vi "GE TRIALNEW 25.vi"() -> ()   [LabVIEW 2014]
uses:
  <vilib>/LabVIEW Targets/FPGA/cRIO/shared/nicrio_ModuleControls/nicrio_cRIO-9225_DataRatesRing.ctl
  <vilib>/LabVIEW Targets/FPGA/cRIO/shared/nicrio_ModuleControls/nicrio_cRIO-9227_DataRatesRing.ctl
  <vilib>/rvi/FXPMathLib/FxpSinAndCos/subVIs/nifxpmath_SinAndCos_SimConfig.ctl
  <vilib>/rvi/FXPMathLib/FxpRectToPolar/subVIs/nifxpmath_RectToPolar_SimConfig.ctl
  <vilib>/rvi/FXPMathLib/FxpDiv/subVIs/nifxpmath_Div_SimConfig.ctl
  <vilib>/rvi/Emulation/niFpgaGetClockAttributes.vi
  <vilib>/rvi/Emulation/niFpgaSctlEmulationGetInTimedLoop.vi
  <vilib>/rvi/Emulation/niFpgaEmulationReportErrorSimple.vi
  <vilib>/rvi/eio/common/nirviEmuTemplateMethod_errors.vi
  <vilib>/rvi/Memory/Memory_Emulation/nirvimemoryFastEmulation.vi
  <vilib>/rvi/Memory/Memory_Emulation/nirvimemoryEmulation.vi
  <vilib>/rvi/Emulation/niFpgaEmulationIsFPGAContextNoSignature.vi
  <vilib>/rvi/DataTransferAndStorage/Container/Common/niFpgaContainerGetUniqueNameForEmu.vi
  <vilib>/rvi/Emulation/niFpgaProcessEmulError.vi
  <vilib>/rvi/errors/nirviReportUnexpectedCaseInternalError (U32).vi
  <vilib>/rvi/FXPMathLib/FxpSinAndCos/simVIs/DllFxpSinAndCosTemp_sub.vi
  <vilib>/rvi/FXPMathLib/FxpRectToPolar/simVIs/DllFxpRectToPolarTemp_sub.vi
  <vilib>/rvi/FXPMathLib/FxpDiv/simVIs/DllFxpDivTemp_sub.vi
  <vilib>/rvi/Emulation/niFpgaCriticalErrorInLSC.vi
  <vilib>/rvi/DataTransferAndStorage/Container/Common/niFpgaContainerSetEmuInfo.vi
  <vilib>/rvi/eio/common/nirviEmuReportErrorAndStop.vi
  <vilib>/rvi/eio/common/nirviEmuTemplatePropertySet_noerrors.vi
  <vilib>/eio/EIONode/EIONode.xnode
  <vilib>/rvi/DataTransferAndStorage/Container/XNode/niFpgaContainer.xnode
  <vilib>/rvi/FXPMathLib/FxpSub/XNode/nifxpmath_Sub.xnode
  <vilib>/rvi/FXPMathLib/FxpMul/XNode/nifxpmath_Multiplier.xnode
  <vilib>/rvi/FXPMathLib/FxpSinAndCos/XNode/nifxpmath_SinAndCos.xnode
  <vilib>/rvi/FXPMathLib/FxpAdd/XNode/nifxpmath_Add.xnode
  <vilib>/rvi/FXPMathLib/FxpRectToPolar/XNode/nifxpmath_RectToPolar.xnode
  <vilib>/rvi/FXPMathLib/FxpDiv/XNode/nifxpmath_Div.xnode
  <vilib>/rvi/LocalResourceManager/LocalResourceManager.xnode
  <vilib>/eio/EIOPropertyNode/EIOPropertyNode.xnode
  <vilib>/rvi/FXPMathLib/sim/FxpSim.dll
  <vilib>/rvi/eio/common/nirviEmuTemplatePropertyGet_errors.vi
  <vilib>/rvi/eio/common/nirviEmuTemplatePropertyGet_noerrors.vi
  <vilib>/rvi/eio/common/nirviEmuTemplatePropertySet_errors.vi
panel:
  in  "stop":bool
  out "Angle Actual":fxp<+/-,22,10>[](array[numeric])
  out "Magnitude Actual":fxp<+,52,38>[](array[numeric])
  out "Ym Magnitude":fxp<+/-,64,39>[](array[numeric])
  out "Ym Angle":fxp<+/-,22,10>[](array[numeric])
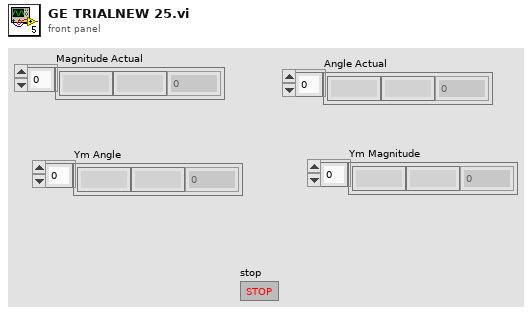
[diagram p1: front panel]
types:
  T1 = typedef "nicrio_cRIO-9227_DataRatesRing.ctl" = u8
  T2 = typedef "nicrio_cRIO-9225_DataRatesRing.ctl" = u8
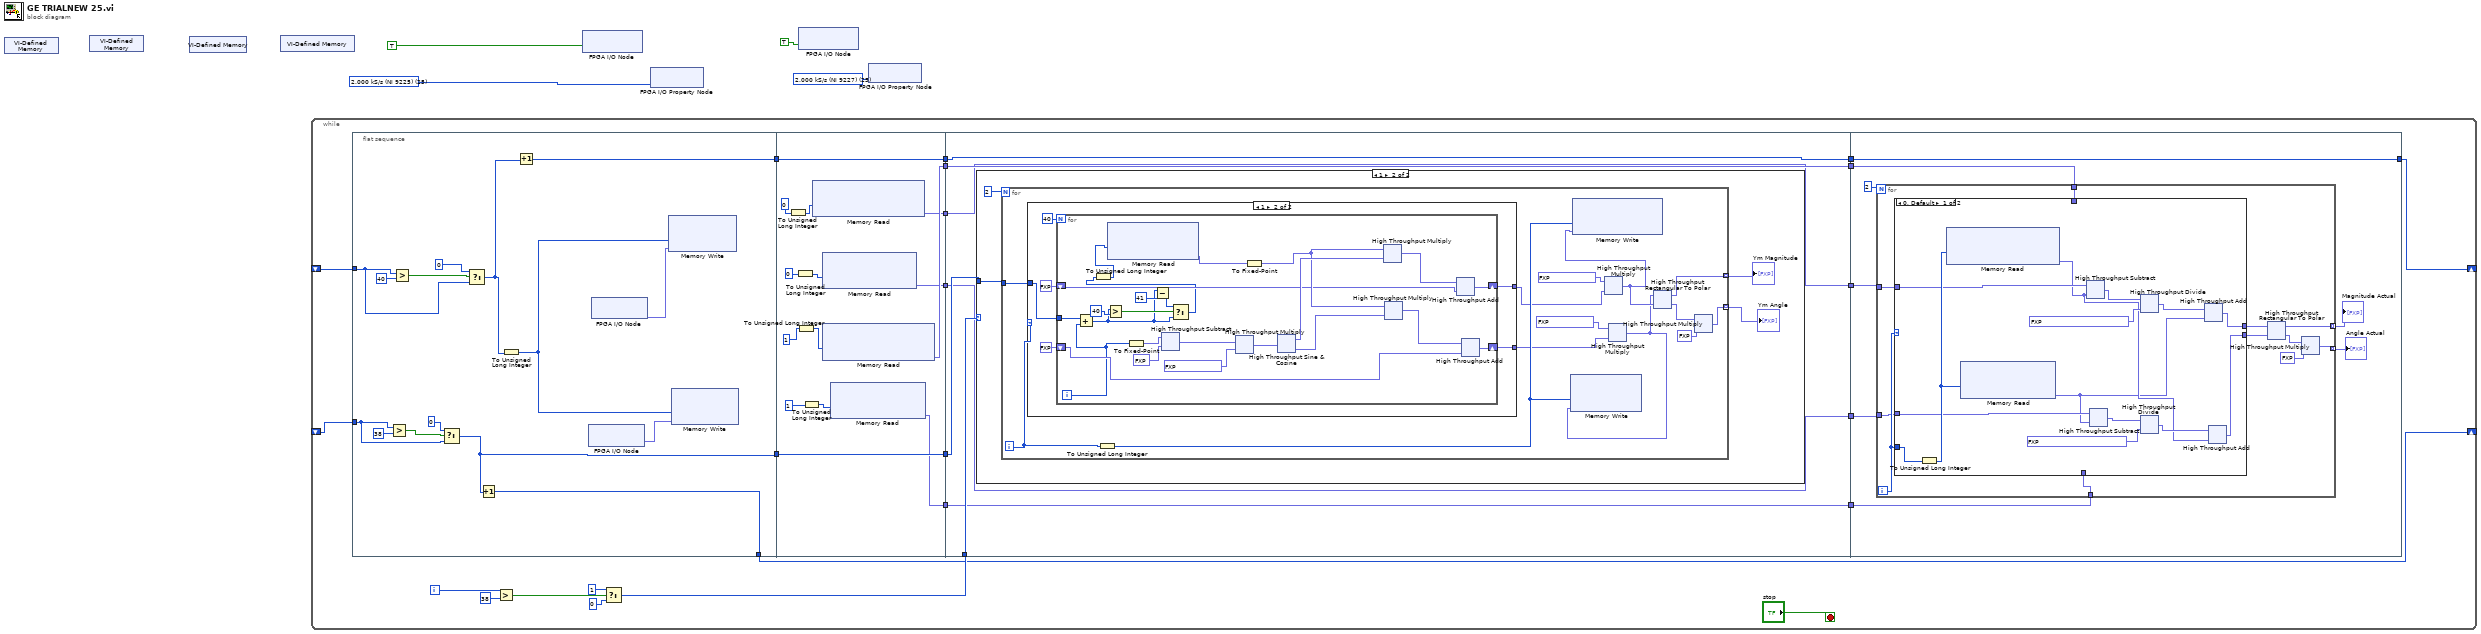
[diagram p0: block diagram]
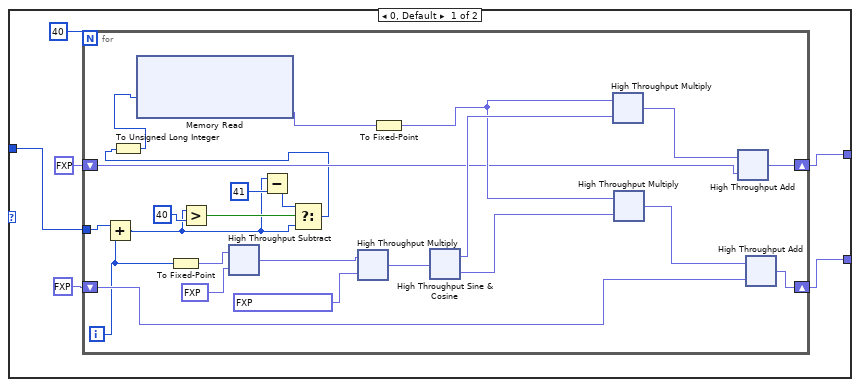
[diagram p3: hidden frame]
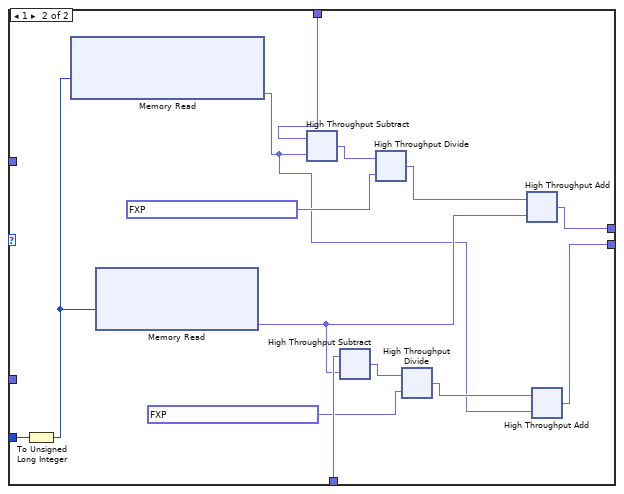
[diagram p4: hidden frame]
diagram:
  w1 = T1 25 items=["50.000 kS/s (NI 9227)"=1, "25.000 kS/s (NI 9227)"=2, "16.667 kS/s (NI 9227)"=3, "12.500 kS/s (NI 9227)"=4, "10.000 kS/s (NI 9227)"=5, "8.333 kS/s (NI 9227)"=6, "7.143 kS/s (NI 9227)"=7, "6.250 kS/s (NI 9227)"=8, "5.556 kS/s (NI 9227)"=9, "5.000 kS/s (NI 9227)"=10, "4.545 kS/s (NI 9227)"=11, "4.167 kS/s (NI 9227)"=12, "3.846 kS/s (NI 9227)"=13, "3.571 kS/s (NI 9227)"=14, "3.333 kS/s (NI 9227)"=15, "3.125 kS/s (NI 9227)"=16, "2.941 kS/s (NI 9227)"=17, "2.778 kS/s (NI 9227)"=18, "2.632 kS/s (NI 9227)"=19, "2.500 kS/s (NI 9227)"=20, "2.381 kS/s (NI 9227)"=21, "2.273 kS/s (NI 9227)"=22, "2.174 kS/s (NI 9227)"=23, "2.083 kS/s (NI 9227)"=24, "2.000 kS/s (NI 9227)"=25, "1.923 kS/s (NI 9227)"=26, "1.852 kS/s (NI 9227)"=27, "1.786 kS/s (NI 9227)"=28, "1.724 kS/s (NI 9227)"=29, "1.667 kS/s (NI 9227)"=30, "1.613 kS/s (NI 9227)"=31] ("Data Rate")
  w2 = T2 25 items=["50.000 kS/s (NI 9225)"=1, "25.000 kS/s (NI 9225)"=2, "16.667 kS/s (NI 9225)"=3, "12.500 kS/s (NI 9225)"=4, "10.000 kS/s (NI 9225)"=5, "8.333 kS/s (NI 9225)"=6, "7.143 kS/s (NI 9225)"=7, "6.250 kS/s (NI 9225)"=8, "5.556 kS/s (NI 9225)"=9, "5.000 kS/s (NI 9225)"=10, "4.545 kS/s (NI 9225)"=11, "4.167 kS/s (NI 9225)"=12, "3.846 kS/s (NI 9225)"=13, "3.571 kS/s (NI 9225)"=14, "3.333 kS/s (NI 9225)"=15, "3.125 kS/s (NI 9225)"=16, "2.941 kS/s (NI 9225)"=17, "2.778 kS/s (NI 9225)"=18, "2.632 kS/s (NI 9225)"=19, "2.500 kS/s (NI 9225)"=20, "2.381 kS/s (NI 9225)"=21, "2.273 kS/s (NI 9225)"=22, "2.174 kS/s (NI 9225)"=23, "2.083 kS/s (NI 9225)"=24, "2.000 kS/s (NI 9225)"=25, "1.923 kS/s (NI 9225)"=26, "1.852 kS/s (NI 9225)"=27, "1.786 kS/s (NI 9225)"=28, "1.724 kS/s (NI 9225)"=29, "1.667 kS/s (NI 9225)"=30, "1.613 kS/s (NI 9225)"=31] ("Data Rate")
  n1 = xnode "VI-Defined Memory"() -> ()  [unwired: 1 out]
  n2 = xnode "VI-Defined Memory"() -> ()  [unwired: 1 out]
  n3 = xnode "VI-Defined Memory"() -> ()  [unwired: 1 out]
  n4 = xnode "VI-Defined Memory"() -> ()  [unwired: 1 out]
  n5 = while {
    shift-right: [w21] -> _
    shift-left: _ -> [w22]
    shift-right: [w18] -> _
    shift-left: _ -> [w19]
    i -> [w25]
    stop <- "stop" stop-if-true
    n6 = flat-sequence {
      tunnel: w22 -> [w35]
      tunnel: [w37] -> w16
      tunnel: w19 -> [w31]
      tunnel: [w30] -> w18
      tunnel: [w29] -> w14
      tunnel: w16 -> [w57]
      tunnel: [w57] -> w15
      tunnel: w14 -> [w56]
      tunnel: [w56] -> w13
      tunnel: [w55] -> w11
      tunnel: [w54] -> w9
      tunnel: [w53] -> w7
      tunnel: [w52] -> w5
      tunnel: w23 -> [w64]
      tunnel: w15 -> [w63]
      tunnel: w13 -> [w62]
      tunnel: [w63] -> w17
      tunnel: [w61] -> w12
      tunnel: w11 -> [w61]
      tunnel: [w60] -> w10
      tunnel: w9 -> [w60]
      tunnel: [w59] -> w8
      tunnel: w7 -> [w59]
      tunnel: [w58] -> w6
      tunnel: w5 -> [w58]
      tunnel: [w246] -> w21
      tunnel: w17 -> [w246]
      tunnel: w12 -> [w244]
      tunnel: w10 -> [w243]
      tunnel: w8 -> [w242]
      tunnel: w6 -> [w241]
      frame #0 {
        n7 = Greater?(x=w31, y=38) -> (0:w32:bool)
        n8 = Greater?(x=w35, y=40) -> (0:w42:bool)
        n9 = Select(t=0, s=w32, f=w31) -> (s? t:f=w29:i32)
        n10 = Select(t=0, s=w42, f=w35) -> (s? t:f=w38:i32)
        n11 = Increment(x=w29) -> (x+1=w30:i32)
        n12 = To Unsigned Long Integer(number=w38) -> (unsigned 32bit integer=w41:u32)
        n13 = Increment(x=w38) -> (x+1=w37:i32)
        n14 = xnode "FPGA I/O Node"() -> ("Mod1/AI0"=w40:fxp<+/-,24,10>)  [unwired: 1 in, 1 out]
        n15 = xnode "FPGA I/O Node"() -> ("Mod2/AI0"=w39:fxp<+/-,24,5>)  [unwired: 1 in, 1 out]
        n16 = xnode ("Memory Write")("Address"=w41, "Data"=w39) -> ()  [unwired: 1 in, 1 out]
        n17 = xnode ("Memory Write")("Address"=w41, "Data"=w40) -> ()  [unwired: 1 in, 1 out]
      }
      frame #1 {
        n18 = To Unsigned Long Integer(number=u32 0 ("Address")) -> (unsigned 32bit integer=w50:u32)
        n19 = To Unsigned Long Integer(number=u32 0 ("Address")) -> (unsigned 32bit integer=w48:u32)
        n20 = To Unsigned Long Integer(number=u32 1 ("Address")) -> (unsigned 32bit integer=w46:u32)
        n21 = To Unsigned Long Integer(number=u32 1 ("Address")) -> (unsigned 32bit integer=w44:u32)
        n22 = xnode ("Memory Read")("Address"=w50) -> ("Data"=w53:fxp<+/-,25,11>)  [unwired: 1 in, 1 out]
        n23 = xnode ("Memory Read")("Address"=w48) -> ("Data"=w52:fxp<+/-,25,11>)  [unwired: 1 in, 1 out]
        n24 = xnode ("Memory Read")("Address"=w46) -> ("Data"=w55:fxp<+/-,25,11>)  [unwired: 1 in, 1 out]
        n25 = xnode ("Memory Read")("Address"=w44) -> ("Data"=w54:fxp<+/-,25,11>)  [unwired: 1 in, 1 out]
      }
      frame #2 {
        n26 = case shown="1" w64 {
          tunnel: w62 -> [_ w67]
          frame 0, Default {
          }
          frame 1 {
            n27 = for {
              N: 2 -> [_]
              tunnel: w67 -> [w81]
              tunnel: [w76] -> w66 mode=indexing
              tunnel: [w75] -> w65 mode=indexing
              i -> [w80]
              n28 = case shown="1" w80 {
                tunnel: w81 -> [w121 w181]
                tunnel: [w120 w180] -> w73
                tunnel: [w119 w179] -> w71
                frame 0, Default {
                  n29 = for {
                    N: 40 -> [_]
                    shift-right: [w136] -> w120
                    shift-left: fxp<+/-,64,37> 0.0 ("x+y") -> [w135]
                    shift-right: [w134] -> w119
                    shift-left: fxp<+/-,45,17> 0.0 ("x+y") -> [w133]
                    tunnel: w121 -> [w131]
                    i -> [w132]
                    n30 = Add(x=w131, y=w132) -> (x+y=w125:i32)
                    n31 = To Fixed-Point(number=w132) -> (fixed-point=w148:fxp<+/-,32,32>)  [unwired: 1 in]
                    n32 = Greater?(x=w125, y=40) -> (0:w129:bool)
                    n33 = xnode "High Throughput Subtract"("x"=w148, "y"=fxp<+,6,5> 19.5) -> ("x-y"=w145:fxp<+/-,34,33>)
                    n34 = Subtract(x=w125, y=41) -> (x-y=w127:i32)
                    n35 = Select(t=w127, s=w129, f=w125) -> (s? t:f=w126:i32)
                    n36 = To Unsigned Long Integer(number=w126) -> (unsigned 32bit integer=w139:u32)
                    n37 = xnode ("Memory Read")("Address"=w139) -> ("Data"=w138:fxp<+/-,25,11>)  [unwired: 1 in, 1 out]
                    n38 = xnode ("High Throughput Multiply")("x"=w145, "y"=fxp<+/-,16,1> 0.04998779296875) -> ("x*y"=w144:fxp<+/-,50,34>)
                    n39 = To Fixed-Point(number=w138) -> (fixed-point=w137:fxp<+/-,25,11>)  [unwired: 1 in]
                    n40 = xnode "High Throughput Sine & Cosine"("x (pi)"=w144) -> ("sin(x)"=w143:fxp<+/-,16,2>, "cos(x)"=w142:fxp<+/-,16,2>)
                    n41 = xnode ("High Throughput Multiply")("x"=w137, "y"=w143) -> ("x*y"=w141:fxp<+/-,41,13>)
                    n42 = xnode ("High Throughput Multiply")("x"=w137, "y"=w142) -> ("x*y"=w140:fxp<+/-,41,13>)
                    n43 = xnode ("High Throughput Add")("x"=w141, "y"=w135) -> ("x+y"=w136:fxp<+/-,64,37>)
                    n44 = xnode ("High Throughput Add")("x"=w140, "y"=w133) -> ("x+y"=w134:fxp<+/-,45,17>)
                  }
                }
                frame 1 {
                  n45 = for {
                    N: 40 -> [_]
                    shift-right: [w196] -> w180
                    shift-left: fxp<+/-,64,37> 0.0 ("x+y") -> [w194]
                    shift-right: [w195] -> w179
                    shift-left: fxp<+/-,45,17> 0.0 ("x+y") -> [w193]
                    tunnel: w181 -> [w191]
                    i -> [w192]
                    n46 = Add(x=w191, y=w192) -> (x+y=w186:i32)
                    n47 = Greater?(x=w186, y=40) -> (0:w189:bool)
                    n48 = To Fixed-Point(number=w192) -> (fixed-point=w208:fxp<+/-,32,32>)  [unwired: 1 in]
                    n49 = Subtract(x=w186, y=41) -> (x-y=w187:i32)
                    n50 = xnode "High Throughput Subtract"("x"=w208, "y"=fxp<+,6,5> 19.5) -> ("x-y"=w205:fxp<+/-,34,33>)
                    n51 = Select(t=w187, s=w189, f=w186) -> (s? t:f=w185:i32)
                    n52 = To Unsigned Long Integer(number=w185) -> (unsigned 32bit integer=w199:u32)
                    n53 = xnode ("Memory Read")("Address"=w199) -> ("Data"=w198:fxp<+/-,25,11>)  [unwired: 1 in, 1 out]
                    n54 = xnode ("High Throughput Multiply")("x"=w205, "y"=fxp<+/-,16,1> 0.04998779296875) -> ("x*y"=w204:fxp<+/-,50,34>)
                    n55 = To Fixed-Point(number=w198) -> (fixed-point=w197:fxp<+/-,25,11>)  [unwired: 1 in]
                    n56 = xnode "High Throughput Sine & Cosine"("x (pi)"=w204) -> ("sin(x)"=w203:fxp<+/-,16,2>, "cos(x)"=w202:fxp<+/-,16,2>)
                    n57 = xnode ("High Throughput Multiply")("x"=w197, "y"=w203) -> ("x*y"=w201:fxp<+/-,41,13>)
                    n58 = xnode ("High Throughput Multiply")("x"=w197, "y"=w202) -> ("x*y"=w200:fxp<+/-,41,13>)
                    n59 = xnode ("High Throughput Add")("x"=w201, "y"=w194) -> ("x+y"=w196:fxp<+/-,64,37>)
                    n60 = xnode ("High Throughput Add")("x"=w200, "y"=w193) -> ("x+y"=w195:fxp<+/-,45,17>)
                  }
                }
              }
              n61 = To Unsigned Long Integer(number=w80) -> (unsigned 32bit integer=w79:u32)
              n62 = xnode ("High Throughput Multiply")("x"=fxp<+/-,16,1> 0.03533935546875 ("y"), "y"=w73) -> ("x*y"=w70:fxp<+/-,64,38>)
              n63 = xnode ("Memory Write")("Address"=w79, "Data"=w70) -> ()  [unwired: 1 in, 1 out]
              n64 = xnode ("High Throughput Multiply")("x"=fxp<+/-,16,1> 0.03533935546875 ("y"), "y"=w71) -> ("x*y"=w69:fxp<+/-,61,18>)
              n65 = xnode ("Memory Write")("Address"=w79, "Data"=w69) -> ()  [unwired: 1 in, 1 out]
              n66 = xnode "High Throughput Rectangular To Polar"("x"=w69, "y"=w70) -> ("magnitude"=w75:fxp<+,64,38>, "phase (pi)"=w77:fxp<+/-,16,2>)
              n67 = xnode ("High Throughput Multiply")("x"=w77, "y"=fxp<+,6,8> 180.0) -> ("x*y"=w76:fxp<+/-,22,10>)
            }
            "Ym Magnitude" <- w65
            "Ym Angle" <- w66
          }
        }
      }
      frame #3 {
        n68 = for {
          N: 2 -> [_]
          tunnel: w244 -> [w256]
          tunnel: w243 -> [w255]
          tunnel: w242 -> [w254]
          tunnel: w241 -> [w253]
          tunnel: [w248] -> w240 mode=indexing
          tunnel: [w247] -> w239 mode=indexing
          i -> [w257]
          n69 = case shown="0, Default" w257 {
            tunnel: w257 -> [w307 w375]
            tunnel: w256 -> [_ w374]
            tunnel: w255 -> [_ w373]
            tunnel: w254 -> [w306 _]
            tunnel: w253 -> [w305 _]
            tunnel: [w296 w364] -> w252
            tunnel: [w295 w363] -> w251
            frame 0, Default {
              n70 = To Unsigned Long Integer(number=w307) -> (unsigned 32bit integer=w308:u32)
              n71 = xnode ("Memory Read")("Address"=w308) -> ("Data"=w298:fxp<+/-,25,11>)  [unwired: 1 in, 1 out]
              n72 = xnode ("Memory Read")("Address"=w308) -> ("Data"=w297:fxp<+/-,25,11>)  [unwired: 1 in, 1 out]
              n73 = xnode "High Throughput Subtract"("x"=w306, "y"=w298) -> ("x-y"=w302:fxp<+/-,26,12>)
              n74 = xnode "High Throughput Subtract"("x"=w305, "y"=w297) -> ("x-y"=w303:fxp<+/-,26,12>)
              n75 = xnode "High Throughput Divide"("x"=w303, "y"=fxp<+,29,4> 12.514757186174393) -> ("x/y"=w299:fxp<+/-,37,37>)
              n76 = xnode "High Throughput Divide"("x"=w302, "y"=fxp<+,29,4> 12.514757186174393) -> ("x/y"=w300:fxp<+/-,37,37>)
              n77 = xnode ("High Throughput Add")("x"=w300, "y"=w297) -> ("x+y"=w296:fxp<+/-,52,38>)
              n78 = xnode ("High Throughput Add")("x"=w299, "y"=w298) -> ("x+y"=w295:fxp<+/-,52,38>)
            }
            frame 1 {
              n79 = To Unsigned Long Integer(number=w375) -> (unsigned 32bit integer=w376:u32)
              n80 = xnode ("Memory Read")("Address"=w376) -> ("Data"=w365:fxp<+/-,25,11>)  [unwired: 1 in, 1 out]
              n81 = xnode ("Memory Read")("Address"=w376) -> ("Data"=w366:fxp<+/-,25,11>)  [unwired: 1 in, 1 out]
              n82 = xnode "High Throughput Subtract"("x"=w374, "y"=w365) -> ("x-y"=w370:fxp<+/-,26,12>)
              n83 = xnode "High Throughput Subtract"("x"=w373, "y"=w366) -> ("x-y"=w369:fxp<+/-,26,12>)
              n84 = xnode "High Throughput Divide"("x"=w370, "y"=fxp<+,29,4> 12.514757186174393) -> ("x/y"=w368:fxp<+/-,37,37>)
              n85 = xnode "High Throughput Divide"("x"=w369, "y"=fxp<+,29,4> 12.514757186174393) -> ("x/y"=w367:fxp<+/-,37,37>)
              n86 = xnode ("High Throughput Add")("x"=w368, "y"=w366) -> ("x+y"=w364:fxp<+/-,52,38>)
              n87 = xnode ("High Throughput Add")("x"=w367, "y"=w365) -> ("x+y"=w363:fxp<+/-,52,38>)
            }
          }
          n88 = xnode "High Throughput Rectangular To Polar"("x"=w252, "y"=w251) -> ("magnitude"=w247:fxp<+,52,38>, "phase (pi)"=w249:fxp<+/-,16,2>)
          n89 = xnode ("High Throughput Multiply")("x"=w249, "y"=fxp<+,6,8> 180.0) -> ("x*y"=w248:fxp<+/-,22,10>)
        }
        "Angle Actual" <- w240
        "Magnitude Actual" <- w239
      }
    }
    n90 = Greater?(x=w25, y=38) -> (0:w26:bool)
    n91 = Select(t=1, s=w26, f=0) -> (s? t:f=w23:i32)
  }
  n92 = xnode "FPGA I/O Node"("Mod1/Start"=TRUE) -> ()  [unwired: 1 in, 1 out]
  n93 = xnode "FPGA I/O Property Node"("Data Rate"=w2) -> ()  [unwired: 1 in, 1 out]
  n94 = xnode "FPGA I/O Node"("Mod2/Start"=TRUE) -> ()  [unwired: 1 in, 1 out]
  n95 = xnode "FPGA I/O Property Node"("Data Rate"=w1) -> ()  [unwired: 1 in, 1 out]
